vi "Factory.vi"(8 "error in (no error)":errorcluster, 10 "Position":cluster{"Row":i8, "Column":i8}, 11 "Type":string) -> (0 "error out":errorcluster, 3 "Amphipod":refnum<class "Amphipod.lvclass">)   [LabVIEW 2019, in "23.lvlib" / "Amphipod.lvclass"]
uses:
  Amphipod.lvclass
  Amber/Amber.lvclass
  C:/Users/craig.walker/Documents/GitHub/lv2019-Advent-of-Code-2021/23/Amphipod/Amphipod.lvclass
  Bronze/Bronze.lvclass
  Copper/Copper.lvclass
  Desert/Desert.lvclass
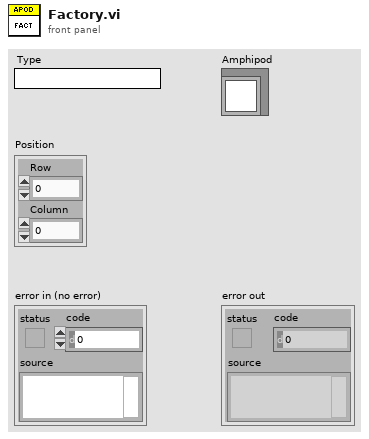
[diagram p1: front panel]
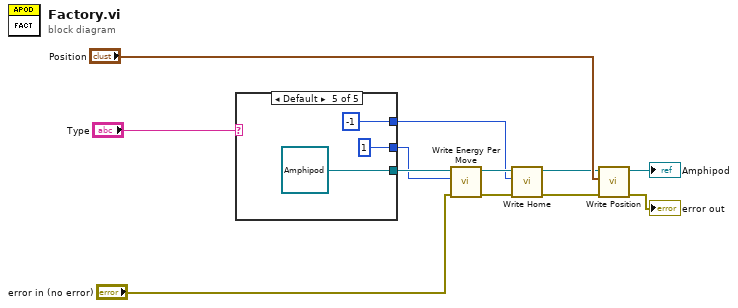
[diagram p0: block diagram]
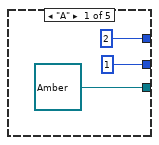
[diagram p2: hidden frame]
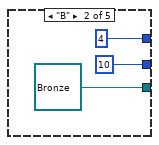
[diagram p3: hidden frame]
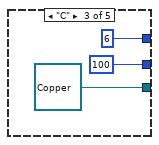
[diagram p4: hidden frame]
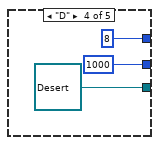
[diagram p5: hidden frame]
diagram:
  n1 = case shown="Default" "Type" {
    tunnel: [refnum<class "Amber.lvclass"> refnum ("23.lvlib:Amber.lvclass") refnum<class "Bronze.lvclass"> refnum ("23.lvlib:Bronze.lvclass") refnum<class "Copper.lvclass"> refnum ("23.lvlib:Copper.lvclass") refnum<class "Desert.lvclass"> refnum ("23.lvlib:Desert.lvclass") refnum<class "Amphipod.lvclass"> refnum ("23.lvlib:Amphipod.lvclass")] -> w12
    tunnel: [u16 1 ("Energy Per Move") u16 10 ("Energy Per Move") u16 100 ("Energy Per Move") u16 1000 ("Energy Per Move") u16 1 ("Energy Per Move")] -> w11
    tunnel: [i8 2 ("Home") i8 4 ("Home") i8 6 ("Home") i8 8 ("Home") i8 -1 ("Home")] -> w1
    frame "A" {
    }
    frame "B" {
    }
    frame "C" {
    }
    frame "D" {
    }
    frame Default {
    }
  }
  n2 = call-dynamic "Write Energy Per Move.vi"("error in (no error)"="error in (no error)", "Energy Per Move"=w11, "Amphipod in"=w12) -> ("error out"=w3:errorcluster, "Amphipod out"=w5:refnum<class "Amphipod.lvclass">)  [unwired: 7 in]
  n3 = call-dynamic "Write Home.vi"("error in (no error)"=w3, "Home"=w1, "Amphipod in"=w5) -> ("error out"=w4:errorcluster, "Amphipod out"=w6:refnum<class "Amphipod.lvclass">)  [unwired: 7 in]
  n4 = call-dynamic "Write Position.vi"("error in (no error)"=w4, "Position"="Position", "Amphipod in"=w6) -> ("error out"=→"error out":errorcluster, "Amphipod out"=→"Amphipod":refnum<class "Amphipod.lvclass">)  [unwired: 7 in]
